vi "Draw Terminals.vi"(6 "State":T2, 7 "Sizes":T1, 11 "Picture  In":picture) -> (3 "Picture":picture)   [LabVIEW 2020, in "FlexBlock.xnode"]
uses:
  FlexBlock.xnode
  State.ctl
  FlexBlocks/Type Descriptor.ctl
  FlexBlocks/Terminal Direction.ctl
  FlexBlocks/Value Mode.ctl
  FlexBlocks/Terminal State.ctl
  FlexBlocks/Special Terminal.ctl
  FlexBlocks/Errors.ctl
  <vilib>/picture/picture.llb/imagedata.ctl
  FlexBlocks/Calculated Sizes.ctl
  FlexBlocks/Size Constants.ctl
  FlexBlocks/FlexBlocks.lvlib
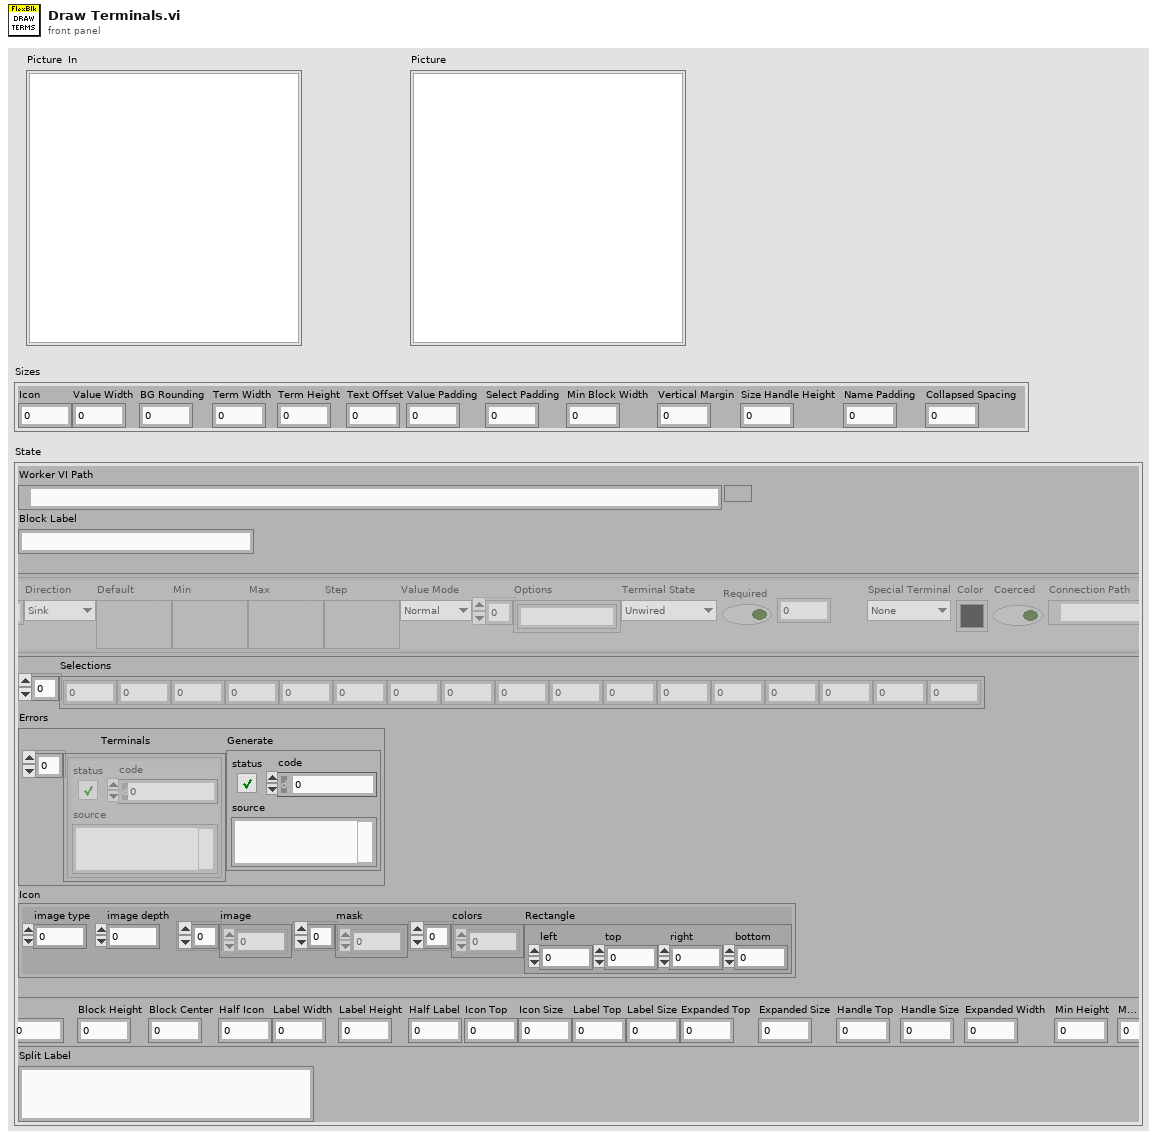
[diagram p1: front panel]
types:
  T1 = typedef "FlexBlocks.lvlib/Size Constants.ctl" = cluster{"Icon":i32, "Value Width":i32, "BG Rounding":i32, "Term Width":i32, "Term Height":i32, "Text Offset":i32, "Value Padding":i32, "Select Padding":i32, "Min Block Width":i32, "Vertical Margin":i32, "Size Handle Height":i32, "Name Padding":i32, "Collapsed Spacing":i32}
  T2 = typedef "FlexBlock.xnode/State.ctl" = cluster{"Worker VI Path":path, "Block Label":string, "Types":T3[], "Selections":i32[], "Errors":T8, "Icon":T9, "Calcd Sizes":T10, "Split Label":string}
  T3 = typedef "FlexBlocks.lvlib/Type Descriptor.ctl" = cluster{"Name":string, "Direction":T4, "Default":variant, "Min":variant, "Max":variant, "Step":variant, "Value Mode":T5, "Options":string[], "Terminal State":T6, "Required":bool, "Connpane Index":i32, "Special Terminal":T7, "Color":u32, "Coerced":bool, "Connection Path":path, "Draw Style":T6}
  T4 = typedef "FlexBlocks.lvlib/Terminal Direction.ctl" = enum16{"Sink", "Source"}
  T5 = typedef "FlexBlocks.lvlib/Value Mode.ctl" = enum16{"Normal", "Range", "Select"}
  T6 = typedef "FlexBlocks.lvlib/Terminal State.ctl" = enum16{"Unwired", "BadType", "BadRef", "Channel", "Value", "Control Ref"}
  T7 = typedef "FlexBlocks.lvlib/Special Terminal.ctl" = enum16{"None", "Action", "Init", "Tag", "State in", "State out", "Error"}
  T8 = typedef "FlexBlocks.lvlib/Errors.ctl" = cluster{"Terminals":errorcluster[], "Generate":errorcluster}
  T9 = typedef "imagedata.ctl" = cluster{"image type":i32, "image depth":i32, "image":u8[], "mask":u8[], "colors":u32[], "Rectangle":cluster{"left":i16, "top":i16, "right":i16, "bottom":i16}}
  T10 = typedef "FlexBlocks.lvlib/Calculated Sizes.ctl" = cluster{"Text Width":i32, "Text Height":i32, "Half Text":i32, "Block Width":i32, "Block Height":i32, "Block Center":i32, "Half Icon":i32, "Label Width":i32, "Label Height":i32, "Half Label":i32, "Icon Top":i32, "Icon Size":i32, "Label Top":i32, "Label Size":i32, "Expanded Top":i32, "Expanded Size":i32, "Handle Top":i32, "Handle Size":i32, "Expanded Width":i32, "Min Height":i32, "Max Height":i32}
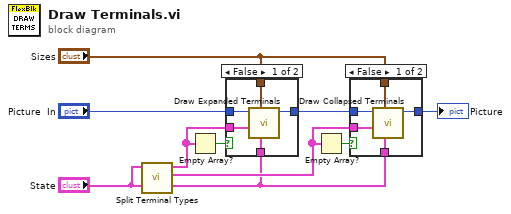
[diagram p0: block diagram]
diagram:
  n1 = call "Split Terminal Types.vi"("State"="State") -> ("Collapsed Types"=w2:T3[], "Expanded Types"=w8:T3[])  [unwired: 9 in]
  n2 = Empty Array?(array=w8) -> (empty?=w7:bool)
  n3 = case shown="False" w7 {
    tunnel: "Picture  In" -> [w14 w15]
    tunnel: [w13 w15] -> w5
    tunnel: "Sizes" -> [w12 _]
    tunnel: "State" -> [w11 _]
    tunnel: w8 -> [w10 _]
    frame False {
      n4 = call "Draw Expanded Terminals.vi"("State"=w11, "Sizes"=w12, "Expanded Types"=w10, "Picture  In"=w14) -> ("Picture"=w13:picture)  [unwired: 7 in]
    }
    frame True {
    }
  }
  n5 = Empty Array?(array=w2) -> (empty?=w6:bool)
  n6 = case shown="False" w6 {
    tunnel: w2 -> [w20 _]
    tunnel: w5 -> [w19 w21]
    tunnel: [w18 w21] -> w4
    tunnel: "Sizes" -> [w17 _]
    tunnel: "State" -> [w16 _]
    frame False {
      n7 = call "Draw Collapsed Terminals.vi"("State"=w16, "Sizes"=w17, "Collapsed Types"=w20, "Picture  In"=w19) -> ("Picture"=w18:picture)  [unwired: 7 in]
    }
    frame True {
    }
  }
  "Picture" <- w4
